vi "CANOpen_READ_PDO_ONLY.vi"() -> ()   [LabVIEW 2017]
uses:
  <vilib>/CANopenLib/CANOPEN.llb/CANopen BaudRate.ctl
  <vilib>/CANopenLib/CANOPEN.llb/CANopen Interface Create.vi
  <vilib>/CANopenLib/CANOPEN.llb/CANopen TPDO Create.vi
panel:
  in  "node-ID":u8=1
  in  "PDO channel":u8(ring) items=["PDO 1", "PDO 2", "PDO 3", "PDO 4"]
  out "data":u8[](array[numeric])
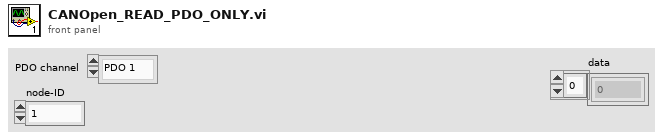
[diagram p1: front panel]
types:
  T1 = typedef "CANopen BaudRate.ctl" = u32
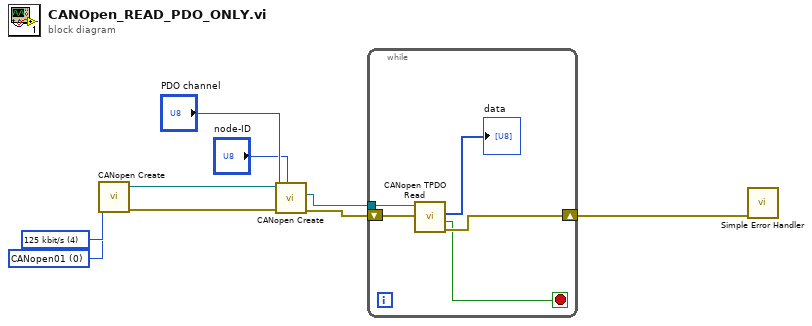
[diagram p0: block diagram]
diagram:
  w8 = u32 0 items=["CANopen01", "CANopen02", "CANopen03", "CANopen04", "CANopen05", "CANopen06", "CANopen07", "CANopen08", "CANopen09", "CANopen10", "CANopen11", "CANopen12", "CANopen13", "CANopen14", "CANopen15", "CANopen16", "CANopen17", "CANopen18", "CANopen19", "CANopen20", "CANopen21", "CANopen22", "CANopen23", "CANopen24", "CANopen25", "CANopen26", "CANopen27", "CANopen28", "CANopen29", "CANopen30", "CANopen31", "CANopen32"] ("interface name")
  w9 = T1 4 items=["1 Mbit/s"=0, "800 kbit/s"=1, "500 kbit/s"=2, "250 kbit/s"=3, "125 kbit/s"=4, "50 kbit/s"=6, "20 kbit/s"=7, "10 kbit/s"=8] ("baud rate")
  n1 = call-poly <vilib>:"CANopen Create.vi"("baud rate"=w9, "interface name"=w8) -> ("error out"=w6:errorcluster, "interface object out"=w7:refnum<k20>)  [unwired: 8 in]
  n2 = call-poly <vilib>:"CANopen Create.vi"("node-ID"="node-ID", "error in (no error)"=w6, "PDO channel"="PDO channel", "interface object in"=w7) -> ("error out"=w4:errorcluster, "TPDO object out"=w5:refnum<k20>)  [unwired: 5 in, 1 out]
  n3 = while {
    tunnel: w5 -> [w14]
    shift-right: [w12] -> w3
    shift-left: w4 -> [w13]
    stop <- w10 stop-if-true
    n4 = call <vilib>:"CANopen TPDO Read.vi"("error in (no error)"=w13, "TPDO object in"=w14) -> ("error out"=w12:errorcluster, "new data?"=w10:bool, "data"=→"data":u8[])  [unwired: 5 in, 2 out]
  }
  n5 = call <vilib>:"Simple Error Handler.vi"("error in (no error)"=w3) -> ()  [unwired: 4 in, 5 out]
